vi "NT Write Raw.vi"(8 "error in":errorcluster, 9 "Raw":string, 11 "Name":string="Raw") -> (0 "error out":errorcluster)   [LabVIEW 2017]
doc: "Write the string to the named entry."
uses:
  <vilib>/Rock Robotics/Network Tables/Field Data.ctl
  <vilib>/Rock Robotics/Network Tables/Field Type.ctl
  <vilib>/Rock Robotics/Network Tables/Sequence.ctl
  <vilib>/Rock Robotics/Network Tables/Write Value Core.vi
  <vilib>/Rock Robotics/Network Tables/Cached Name Lookup.vi
  <vilib>/Rock Robotics/Network Tables/Create Actual Table Name.vi
  <vilib>/Rock Robotics/Network Tables/Manage Dirty Field ID List.vi
  <vilib>/Rock Robotics/Network Tables/NT Globals.vi
  <vilib>/Rock Robotics/Network Tables/Update Other Clients.vi
  <vilib>/Rock Robotics/Network Tables/Build Entry Assign Buffer.vi
  <vilib>/Rock Robotics/Network Tables/Field Data Manager.vi
  <vilib>/Rock Robotics/Network Tables/Usage Statistics.vi
  <vilib>/Rock Robotics/Network Tables/Table Manager.vi
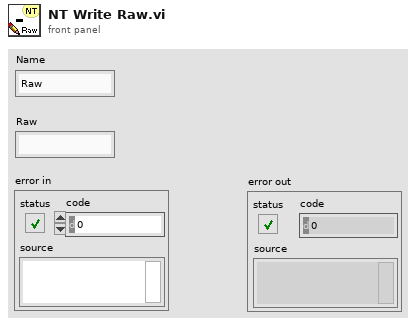
[diagram p1: front panel]
types:
  T1 = typedef "Field Data.ctl" = cluster{"Dbl":dbl, "String":string, "Type":T2, "Boolean":bool, "Sequence #":T3, "Flags":u8}
  T2 = typedef "Field Type.ctl" = enum8{"Invalid", "Bool", "Numeric", "String", "Raw", "Boolean Array", "Numeric Array", "String Array", "RPC"}
  T3 = typedef "Sequence.ctl" = u16
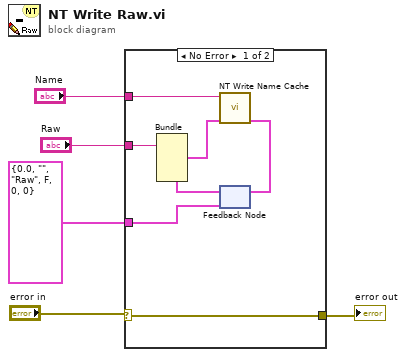
[diagram p0: block diagram]
diagram:
  n1 = case shown="No Error" "error in" {
    selector: "error in" -> [w6 w13]
    tunnel: "Raw" -> [w12 _]
    tunnel: "Name" -> [w10 _]
    tunnel: T1 {"Dbl"=0.0, "String"="", "Type"=enum."Raw", "Boolean"=FALSE, "Sequence #"=0, "Flags"=0} ("Field Value In") -> [w7 _]
    tunnel: [w6 w13] -> w1
    frame No Error {
      n2 = feedback #1(w7) -> (w8:T1)
      n3 = Bundle(cluster=w8, "String"=w12) -> (w11:T1)  [unwired: 5 in]
      n4 = call <vilib>:"NT Write Name Cache.vi"("Field Value In"=w11, "Name"=w10) -> ("Field Value Out"=w9:T1)  [unwired: 9 in]
      n5 = feedback-in #1(w9) -> ()
    }
    frame Error {
    }
  }
  "error out" <- w1
